vi "16.Evd.6_Ask.1_2.vi"() -> ()   [LabVIEW 2020]
uses:
  Control 1.ctl
panel:
  out "x/y":dbl
  in  "Array 5":dbl[](array[numeric])
  out "Array 4":dbl[][](array[numeric])
  out "Array 3":T1[](array[typedef])
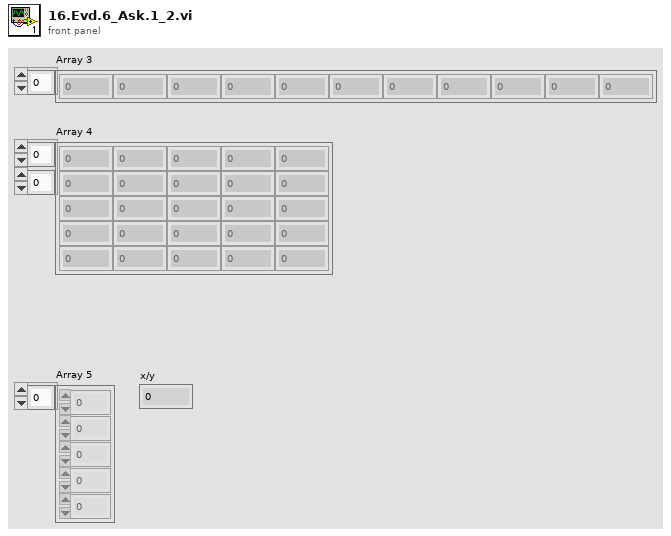
[diagram p1: front panel]
types:
  T1 = typedef "Control 1.ctl" = dbl
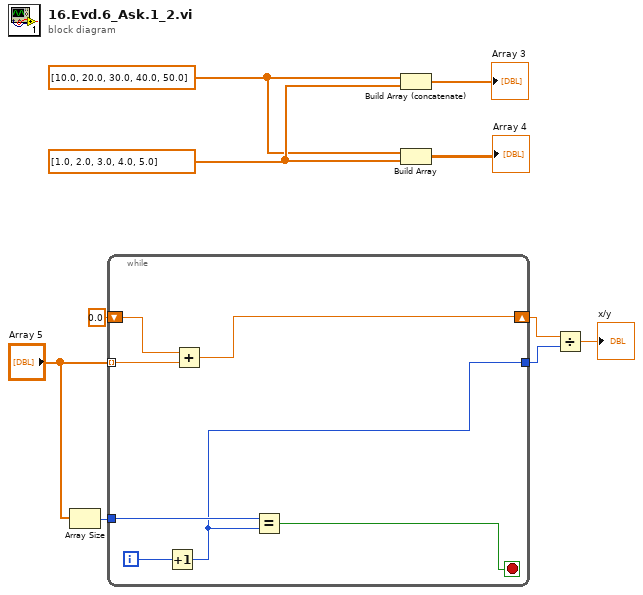
[diagram p0: block diagram]
diagram:
  w1 = dbl[] [10.0, 20.0, 30.0, 40.0, 50.0] ("Array")
  w2 = dbl[] [1.0, 2.0, 3.0, 4.0, 5.0] ("Array 2")
  n1 = Array Size(array="Array 5") -> (size(s)=w3:i32)
  n2 = while {
    tunnel: [w11] -> w8
    shift-right: [w15] -> w6
    shift-left: 0.0 -> [w16]
    tunnel: "Array 5" -> [w17] mode=indexing
    tunnel: w3 -> [w13]
    i -> [w12]
    stop <- w14 stop-if-true
    n3 = Increment(x=w12) -> (x+1=w11:i32)
    n4 = Add(x=w16, y=w17) -> (x+y=w15:dbl)
    n5 = Equal?(x=w13, y=w11) -> (x = y?=w14:bool)
  }
  n6 = Build Array (concatenate)(w1, w2) -> (→"Array 3":dbl[])
  n7 = Build Array(w1, w2) -> (→"Array 4":dbl[][])
  n8 = Divide(x=w6, y=w8) -> (x/y=→"x/y":dbl)
